vi "subsector to sick value.vi"(1 "Subsector":i32[](array[numeric]), 2 "Sick values":i32[](array[numeric])) -> (0 "Subsector sick value":i32)   [LabVIEW 2009]
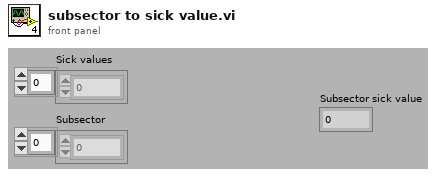
[diagram p1: front panel]
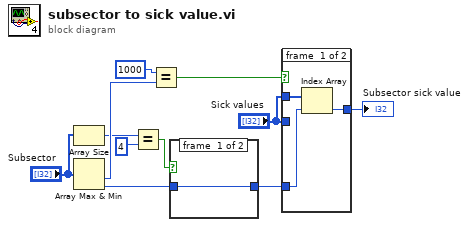
[diagram p0: block diagram]
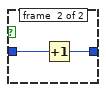
[diagram p2: hidden frame]
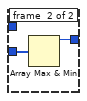
[diagram p3: hidden frame]
diagram:
  n1 = Array Size(array="Subsector") -> (size(s)=w5:i32)
  n2 = Array Max & Min(array="Subsector") -> (min value=w10:i32, min index (indices)=w2:i32)  [unwired: 2 out]
  n3 = Equal?(x=w5, y=4) -> (x = y?=w3:bool)
  n4 = Equal?(x=1000, y=w10) -> (x = y?=w11:bool)
  n5 = case "Since the right camera can see the lowest\nsick value and the left camera can't, we \nmust increase the index of the minmum\nvalue by 1 if we are dealing with the left \ncamera. This ensures that the left camera \nnever sees the lowest sick value by mistake.\nWe check whether we are dealing with the\nright or the left by checking the size of the\nsubsector. The left has 4 subsectors, and\nthe right has 5." shown="True" w3 {
    tunnel: w2 -> [w12 w14]
    tunnel: [w12 w13] -> w1
    frame #0 {
    }
    frame #1 {
      n6 = Increment(x=w14) -> (x+1=w13:i32)
    }
  }
  n7 = case "If the minimum value is 1000, then we assume that\nall values in the subsector are 1000, and we assign\nthe highest possible sick value to that subsector. \n1000 is a somewhat arbitrary number that is \nassigned to all regions which are empty. If the\nminimum value is not 1000, we take the\ncorresponding element of the sick value array and\nuse that s the subsector's sick value." shown="False" w11 {
    tunnel: w1 -> [w17 _]
    tunnel: "Sick values" -> [w16 _]
    tunnel: [w15 w18] -> w8
    tunnel: "Sick values" -> [_ w19]
    frame #0 {
      n8 = Index Array(array=w16, index=w17) -> (element=w15:i32)
    }
    frame #1 {
      n9 = Array Max & Min(array=w19) -> (max value=w18:i32)  [unwired: 3 out]
    }
  }
  "Subsector sick value" <- w8
